vi "Return X Position of Cursors.vi"(11 "WaveformGraph in":refnum<vi>) -> (1 "Cursor 1 X Pos":dbl, 2 "Cursor 2 X Pos":dbl, 3 "Cursor 3 X Pos":dbl)   [LabVIEW 2016]
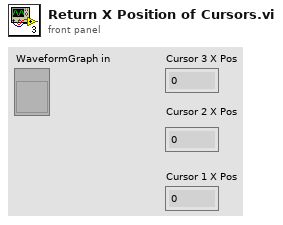
[diagram p1: front panel]
types:
  T1 = typedef "LVCursorListTypeDef.ctl" = cluster{"Name":string, "Color":u32, "Style":u8, "Point Style":u8, "Name Visible":bool, "Allow Drag":bool, "Cursor Mode":u32, "Plot":i32, "Index":i32, "Position":cluster{"X":dbl, "Y":dbl}, "X Scale":u32, "Y Scale":u32, "Watch Plots":i32[], "Watch All Plots":bool, "Plot Area":i32, "Label Offset":cluster{"X":dbl, "Y":dbl}}[]
  T2 = cluster{"Name":string, "Color":u32, "Style":u8, "Point Style":u8, "Name Visible":bool, "Allow Drag":bool, "Cursor Mode":u32, "Plot":i32, "Index":i32, "Position":cluster{"X":dbl, "Y":dbl}, "X Scale":u32, "Y Scale":u32, "Watch Plots":i32[], "Watch All Plots":bool, "Plot Area":i32, "Label Offset":cluster{"X":dbl, "Y":dbl}}
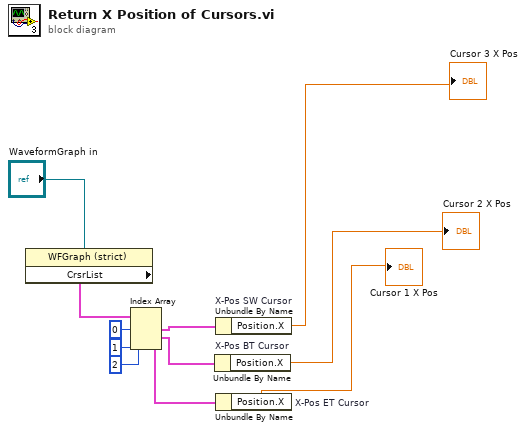
[diagram p0: block diagram]
diagram:
  n1 = property on="Property Node" class="WFGraph (strict)"(reference="WaveformGraph in") -> ("CrsrList"=w1:T1)  [unwired: 1 in, 2 out]
  n2 = Index Array(array=w1, index #1=0 ("index"), index #2=1 ("index"), index #3=2 ("index")) -> (element #1=w6:T2, element #2=w7:T2, element #3=w8:T2)
  n3 = Unbundle By Name "X-Pos BT Cursor"(w7) -> ("Position.X"=→"Cursor 2 X Pos":dbl)
  n4 = Unbundle By Name "X-Pos SW Cursor"(w6) -> ("Position.X"=→"Cursor 3 X Pos":dbl)
  n5 = Unbundle By Name "X-Pos ET Cursor"(w8) -> ("Position.X"=→"Cursor 1 X Pos":dbl)
